vi "list_component_configurations.vi"(7 "progress bar ref":refnum<vi>, 8 "error in (no error)":errorcluster, 10 "user name":string, 11 "tree ref":refnum<vi>) -> (0 "error out":errorcluster)   [LabVIEW 2010]
uses:
  common/classes/ErrorController/ErrorController/class_data.vi
  common/classes/ErrorController/ErrorController/ErrorController.lvclass
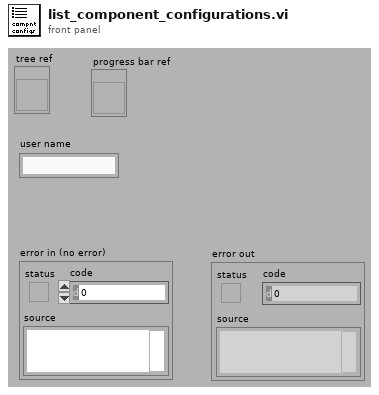
[diagram p1: front panel]
types:
  T1 = typedef "configuration_paths_cluster.ctl" = cluster{"base folder":path, "base folder for user":path, "component folder":path, "component file path":path, "main folder":path, "main file":path}
  T2 = typedef "component_path_clusters.ctl" = cluster{"components directory":path, "component type directory":path, "specific component directory":path, "component class path":path}
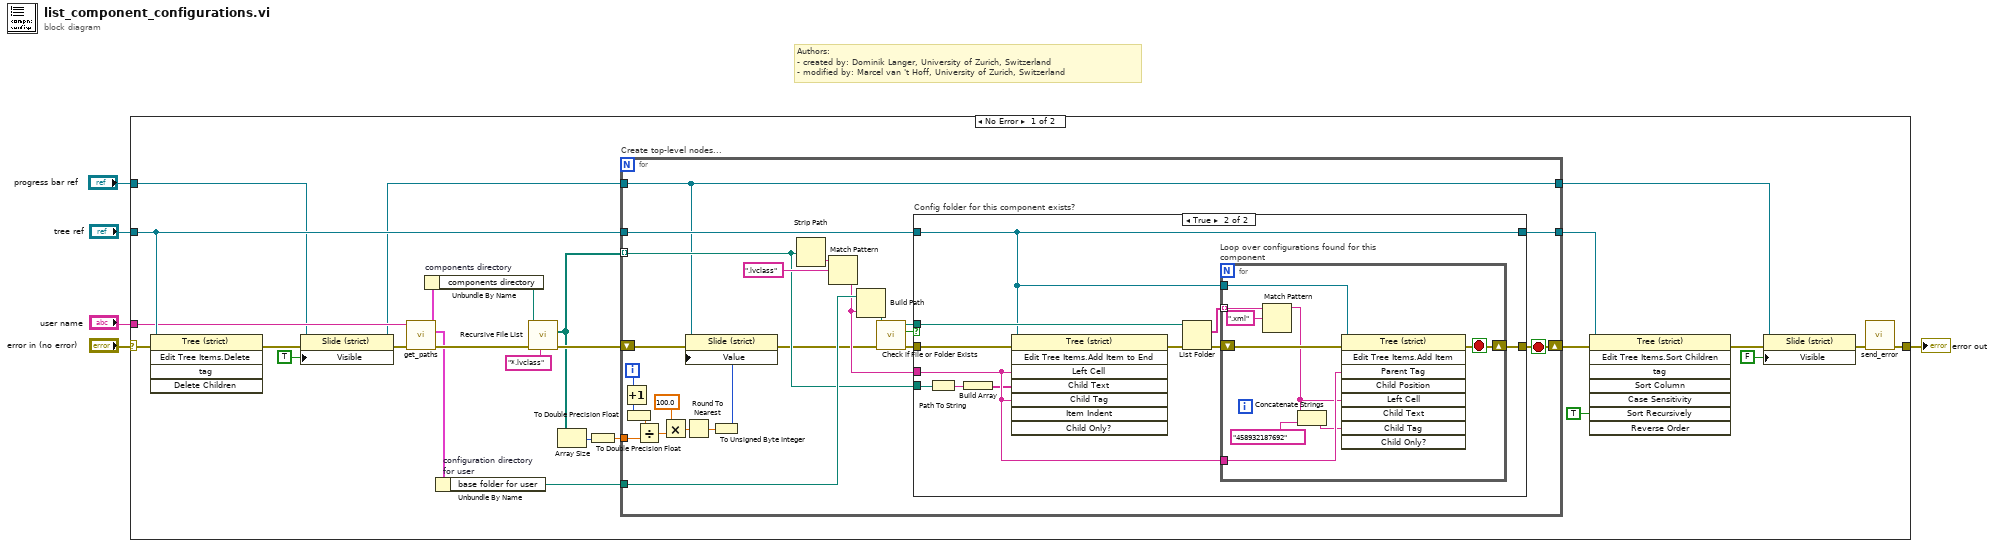
[diagram p0: block diagram]
diagram:
  # "Authors: \n- created by: Dominik Langer, University of Zurich, Switzerland\n- modified by: Marcel van 't Hoff, University of Zurich, Switzerland"
  n1 = case shown="No Error" "error in (no error)" {
    selector: "error in (no error)" -> [w26 w78]
    tunnel: [w6 w78] -> w4
    tunnel: "tree ref" -> [w31 _]
    tunnel: "user name" -> [w22 _]
    tunnel: "progress bar ref" -> [w15 _]
    frame No Error {
      n2 = invoke on="Invoke Node" class="Tree (strict)" method="Edit Tree Items.Delete"(reference=w31, error in=w26) -> (error out=w13:errorcluster)  [unwired: 3 in, 4 out]
      n3 = property class="Slide (strict)"(reference=w15, error in=w13, "Visible"=TRUE) -> (reference out=w14:refnum<vi>, error out=w12:errorcluster)
      n4 = call "get_paths.vi"("error in (no error)"=w12, "user"=w22) -> ("error out"=w25:errorcluster, "configuration paths"=w24:T1, "component paths"=w28:T2)  [unwired: 6 in, 1 out]
      n5 = Unbundle By Name "components directory"(w28) -> ("components directory"=w27:path)
      n6 = Unbundle By Name "configuration directory for user"(w24) -> ("base folder for user"=w23:path)
      n7 = call <vilib>:"Recursive File List.vi"("pattern"="*.lvclass", "error in (no error)"=w25, "Folder Path"=w27) -> ("error out"=w29:errorcluster, "All Files in Dir"=w21:path[])  [unwired: 1 in, 6 out]
      n8 = Array Size(array=w21) -> (size(s)=w20:i32)
      n9 = To Double Precision Float(number=w20) -> (double precision float=w19:dbl)
      n10 = for "Create top-level nodes..." {
        tunnel: w21 -> [w47] mode=indexing
        tunnel: w23 -> [w53]
        tunnel: w31 -> [w46]
        tunnel: w14 -> [w32]
        tunnel: w19 -> [w43]
        tunnel: [w33] -> w17
        tunnel: [w32] -> w8
        shift-right: [w45] -> w18
        shift-left: w29 -> [w42]
        i -> [w34]
        stop <- w45 stop-if-true
        n11 = Increment(x=w34) -> (x+1=w35:i32)
        n12 = To Double Precision Float(number=w35) -> (double precision float=w44:dbl)
        n13 = Divide(x=w44, y=w43) -> (x/y=w40:dbl)
        n14 = Multiply(x=100.0, y=w40) -> (x*y=w38:dbl)
        n15 = Round To Nearest(number=w38) -> (nearest integer value=w37:dbl)
        n16 = To Unsigned Byte Integer(number=w37) -> (unsigned 8bit integer=w36:u8)
        n17 = property class="Slide (strict)"(reference=w32, error in=w42, "Value"=w36) -> (error out=w41:errorcluster)  [unwired: 1 out]
        n18 = Strip Path(path=w47) -> (name=w55:string)  [unwired: 1 out]
        n19 = Match Pattern(string=w55, regular expression=".lvclass") -> (before substring=w49:string)  [unwired: 4 out]
        n20 = Build Path(base path=w53, name or relative path=w49) -> (appended path=w51:path)
        n21 = call <vilib>:"Check if File or Folder Exists.vi"("error in (no error)"=w41, "path"=w51) -> ("error out"=w52:errorcluster, "file or folder exists?"=w48:bool, "dup path"=w50:path)  [unwired: 7 out]
        n22 = case "Config folder for this component exists?" shown="True" w48 {
          tunnel: [w57 w65] -> w45
          tunnel: w52 -> [w57 w64]
          tunnel: w50 -> [_ w63]
          tunnel: w49 -> [_ w59]
          tunnel: w47 -> [_ w62]
          tunnel: w46 -> [w56 w60]
          tunnel: [w56 w60] -> w33
          frame False {
          }
          frame True {
            n23 = Path To String(path=w62) -> (string=w61:string)
            n24 = Build Array(w61) -> (w58:string[])
            n25 = invoke on="Invoke Node" class="Tree (strict)" method="Edit Tree Items.Add Item to End"(reference=w60, error in=w64, "Left Cell"=w59, "Child Text"=w58, "Child Tag"=w59) -> (error out=w66:errorcluster)  [unwired: 3 in, 7 out]
            n26 = List Folder(path=w63, error in=w66) -> (filenames=w68:string[], error out=w67:errorcluster)  [unwired: 4 out]
            n27 = for "Loop over configurations found for this component" {
              tunnel: w68 -> [w76] mode=indexing
              tunnel: w59 -> [w73]
              tunnel: w60 -> [w74]
              shift-right: [w69] -> w65
              shift-left: w67 -> [w77]
              stop <- w69 stop-if-true
              n28 = Match Pattern(string=w76, regular expression=".xml") -> (before substring=w72:string)  [unwired: 4 out]
              n29 = Concatenate Strings(w72, "458932187692") -> (w71:string)
              n30 = invoke on="Invoke Node" class="Tree (strict)" method="Edit Tree Items.Add Item"(reference=w74, error in=w77, "Parent Tag"=w73, "Left Cell"=w72, "Child Tag"=w71) -> (error out=w69:errorcluster)  [unwired: 4 in, 8 out]
            }
          }
        }
      }
      n31 = invoke on="Invoke Node" class="Tree (strict)" method="Edit Tree Items.Sort Children"(reference=w17, error in=w18, "Sort Recursively"=TRUE ("Sort Recursively?")) -> (error out=w9:errorcluster)  [unwired: 5 in, 7 out]
      n32 = property class="Slide (strict)"(reference=w8, error in=w9, "Visible"=FALSE) -> (error out=w7:errorcluster)  [unwired: 1 out]
      n33 = call "send_error.vi"("error in (no error)"=w7) -> ("error out"=w6:errorcluster)  [unwired: 10 in]
    }
    frame Error {
    }
  }
  "error out" <- w4
